vi "Generate Data Frame Vectors.vi"(0 "RFFE RegWrite Command in":refnum<class "RFFE RegWrite Command.lvclass">, 11 "error in (no error)":errorcluster) -> (4 "RFFE RegWrite Command out":refnum<class "RFFE RegWrite Command.lvclass">, 6 "Data Frame Vectors":string[](array[string]), 15 "error out":errorcluster)   [LabVIEW 2018, in "MIPI RFFE API.lvlib" / "RFFE RegWrite Command.lvclass"]
uses:
  RFFE RegWrite Command.lvclass
  MIPI RFFE API.lvlib
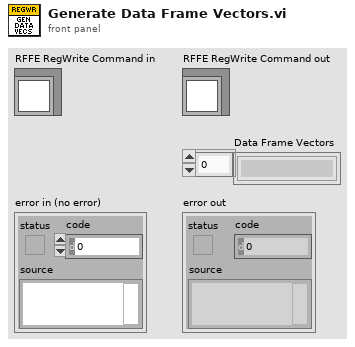
[diagram p1: front panel]
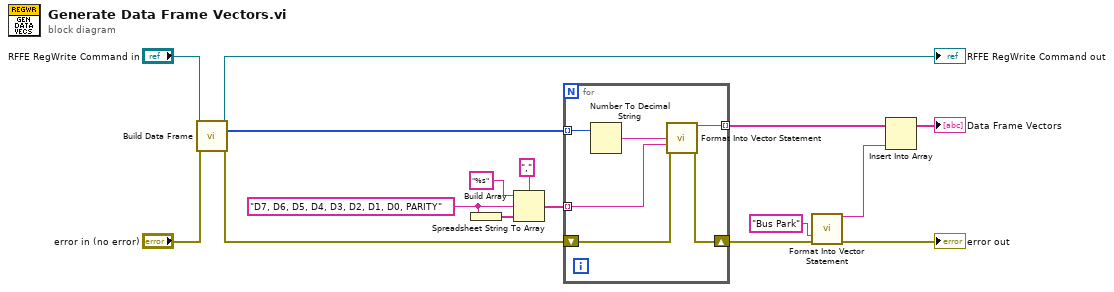
[diagram p0: block diagram]
diagram:
  w13 = "D7, D6, D5, D4, D3, D2, D1, D0, PARITY"
  n1 = call-dynamic "Build Data Frame.vi"("RFFE RegWrite Command in"="RFFE RegWrite Command in", "error in (no error)"="error in (no error)") -> ("RFFE RegWrite Command out"=→"RFFE RegWrite Command out":refnum<class "RFFE RegWrite Command.lvclass">, "Data Frame"=w7:u8[], "error out"=w8:errorcluster)  [unwired: 11 in]
  n2 = Build Array(w13) -> (w12:string[])
  n3 = Spreadsheet String To Array(delimiter (Tab)=",", format string="%s", spreadsheet string=w13, array type (2D Dbl)=w12) -> (array=w9:string[])
  n4 = for {
    tunnel: w7 -> [w22] mode=indexing
    shift-right: [w18] -> w5
    shift-left: w8 -> [w19]
    tunnel: w9 -> [w20] mode=indexing
    tunnel: [w17] -> w3 mode=indexing
    n5 = Number To Decimal String(number=w22) -> (decimal integer string=w21:string)  [unwired: 1 in]
    n6 = call "Format Into Vector Statement.vi"("DATA (0)"=w21, "Comment"=w20, "error in (no error)"=w19) -> ("Vector Statement"=w17:string, "error out"=w18:errorcluster)  [unwired: 11 in]
  }
  n7 = call "Format Into Vector Statement.vi"("Comment"="Bus Park", "error in (no error)"=w5) -> ("Vector Statement"=w1:string, "error out"=→"error out":errorcluster)  [unwired: 12 in]
  n8 = Insert Into Array(array=w3, new element=w1) -> (→"Data Frame Vectors":string[])  [unwired: 1 in]
